vi "releaseShMem.vi"(8 "error in (no error)":errorcluster, 11 "SalProcess in":refnum<class "SalProcess.lvclass">) -> (0 "error out":errorcluster, 2 "function return":i32, 3 "SalProcess out":refnum<class "SalProcess.lvclass">)   [LabVIEW 2018, in "SalProcess.lvclass"]
doc: "Release the shared memory."
uses:
  SalProcess.lvclass
  SalProcess.lvclass/SalProcess.ctl
  LibReader/LibReader.lvclass
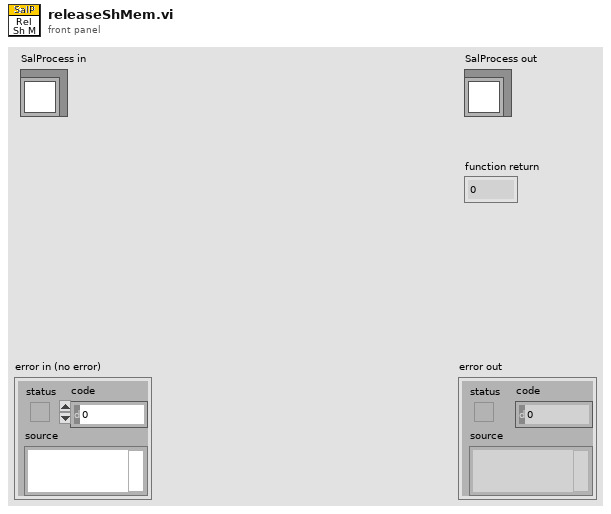
[diagram p1: front panel]
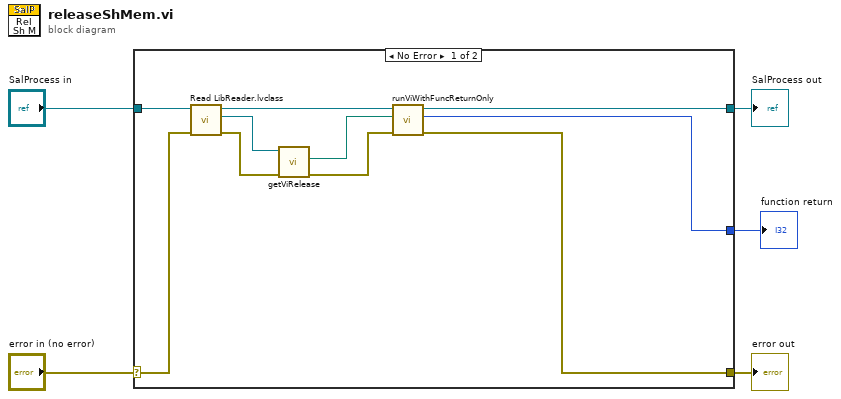
[diagram p0: block diagram]
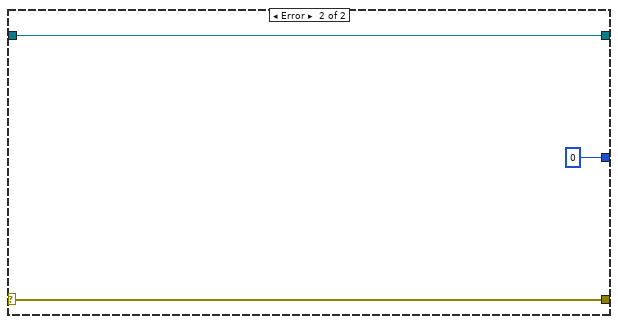
[diagram p2: hidden frame]
diagram:
  n1 = case shown="No Error" "error in (no error)" {
    selector: "error in (no error)" -> [w13 w18]
    tunnel: [w7 w18] -> w4
    tunnel: [w10 w17] -> w2
    tunnel: "SalProcess in" -> [w15 w17]
    tunnel: [w6 0 ("function return")] -> w1
    frame No Error {
      n2 = call "Read LibReader.lvclass.vi"("error in (no error)"=w13, "SalProcess in"=w15) -> ("error out"=w12:errorcluster, "LibReader.lvclass"=w14:refnum<class "LibReader.lvclass">, "SalProcess out"=w11:refnum<class "SalProcess.lvclass">)  [unwired: 7 in]
      n3 = call "getViRelease.vi"("error in (no error)"=w12, "LibReader in"=w14) -> ("error out"=w8:errorcluster, "pathViRelease"=w9:path)  [unwired: 7 in, 1 out]
      n4 = call "runViWithFuncReturnOnly.vi"("error in (no error)"=w8, "vi path"=w9, "SalProcess in"=w11) -> ("error out"=w7:errorcluster, "function return"=w6:i32, "SalProcess out"=w10:refnum<class "SalProcess.lvclass">)  [unwired: 6 in]
    }
    frame Error {
    }
  }
  "error out" <- w4
  "SalProcess out" <- w2
  "function return" <- w1
